vi "Update pump.vi"(5 "new pump cmd":bool, 7 "Pump updates":T1 {"Update Time" format="%.2f"}, 9 "write interval (s)":dbl=5.0, 10 "Time":dbl format="%.2f", 11 "State":i16) -> (3 "update":bool)   [LabVIEW 2019]
uses:
  Pump updates.ctl
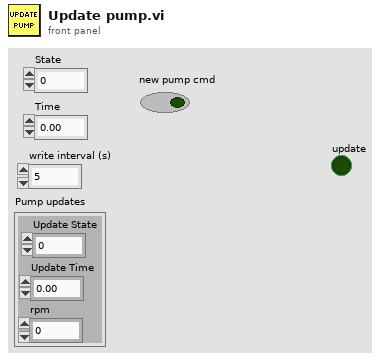
[diagram p1: front panel]
types:
  T1 = typedef "Pump updates.ctl" = cluster{"Update State":i16, "Update Time":dbl, "rpm":dbl}
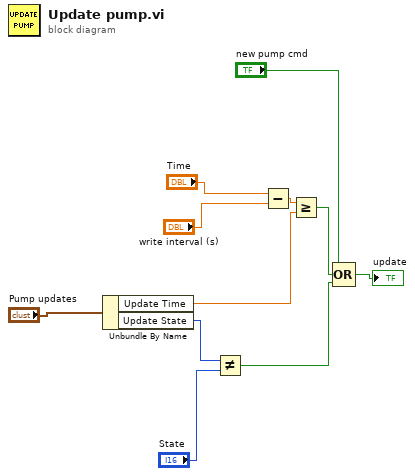
[diagram p0: block diagram]
diagram:
  n1 = Unbundle By Name("Pump updates") -> ("Update Time"=w5:dbl, "Update State"=w4:i16)
  n2 = Not Equal?(x=w4, y="State") -> (x != y?=w7:bool)
  n3 = Subtract(x="Time", y="write interval (s)") -> (x-y=w9:dbl)
  n4 = Greater Or Equal?(x=w9, y=w5) -> (x >= y?=w8:bool)
  n5 = Compound Arithmetic op=OR("new pump cmd", w8, w7) -> (→"update":bool)
